vi "WFPadToEvenSamplesD.vi"(4 "error in (no error)":errorcluster, 7 "Waveform In":digitalwaveform(waveform)={"t0"=timestamp(0 s since 1904-01-01), "dt"=1.0, "Y"={"transitions"=[], "data"=[]}}) -> (0 "error out":errorcluster, 3 "Waveform Out":digitalwaveform(waveform)={"t0"=timestamp(0 s since 1904-01-01), "dt"=1.0, "Y"={"transitions"=[], "data"=[]}})   [LabVIEW 2013]
uses:
  <vilib>/Waveform/DWDTOps.llb/DWDT Digital Size.vi
  <vilib>/Waveform/DWDTOps.llb/DWDT Digital to Boolean Array.vi
  <vilib>/Waveform/DWDTOps.llb/DWDT Boolean Array to Digital.vi
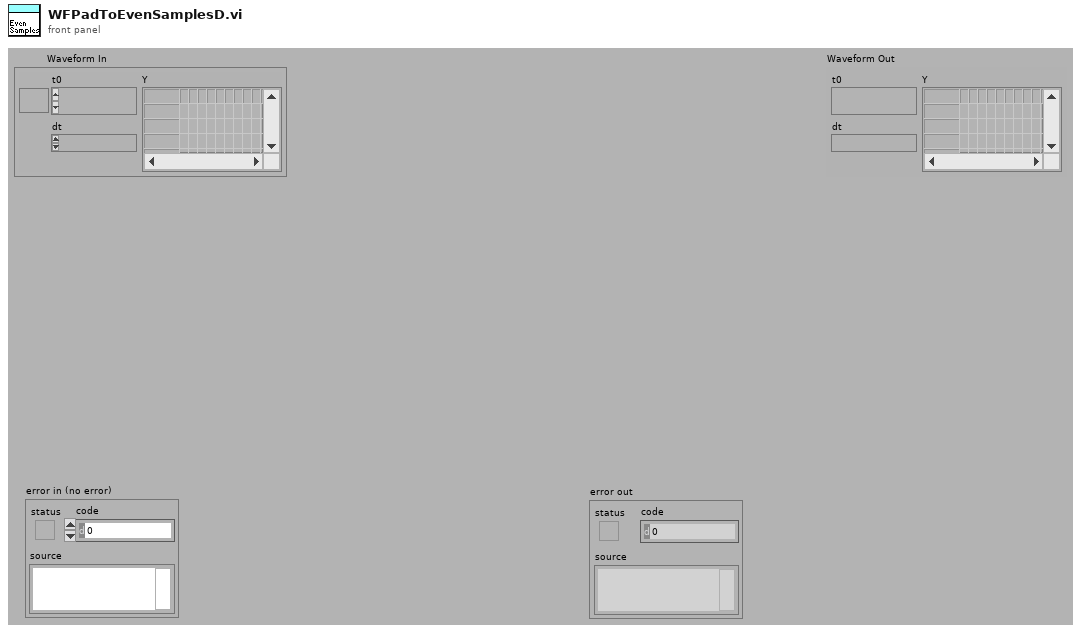
[diagram p1: front panel]
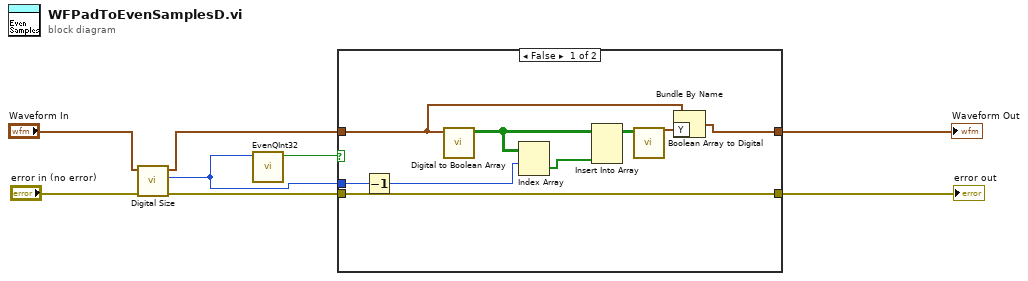
[diagram p0: block diagram]
diagram:
  n1 = call-poly <vilib>:"Digital Size.vi"("error in (no error)"="error in (no error)", "digital waveform in"="Waveform In") -> ("error out"=w2:errorcluster, "number of samples"=w1:i32, "digital waveform out"=w3:digitalwaveform)  [unwired: 6 in, 1 out]
  n2 = call "EvenQInt32.vi"("Input"=w1) -> ("Result"=w7:bool)  [unwired: 10 in]
  n3 = case shown="False" w7 {
    tunnel: w2 -> [w16 w19]
    tunnel: [w16 w19] -> w8
    tunnel: w3 -> [w15 w18]
    tunnel: [w17 w18] -> w6
    tunnel: w1 -> [w11 _]
    frame False {
      n4 = Decrement(x=w11) -> (x-1=w10:i32)
      n5 = call-poly <vilib>:"Digital to Boolean Array.vi"("digital waveform"=w15) -> ("boolean array"=w12:bool[][])  [unwired: 9 in, 1 out]
      n6 = Index Array(array=w12, index (row)=w10) -> (element=w9:bool[])  [unwired: 1 in]
      n7 = Insert Into Array(array=w12, new element=w9) -> (w14:bool[][])  [unwired: 2 in]
      n8 = call-poly <vilib>:"Boolean Array to Digital.vi"("boolean array"=w14) -> ("digital waveform"=w13:digitalwaveform)  [unwired: 9 in, 1 out]
      n9 = Bundle By Name(cluster=w15, "Y"=w13) -> (w17:digitalwaveform)
    }
    frame True {
    }
  }
  "Waveform Out" <- w6
  "error out" <- w8
